vi "ConfigureChannels.vi"(8 "error in (no error)":errorcluster, 11 "Infiniium in":refnum<class "Infiniium.lvclass">) -> (0 "error out":errorcluster, 3 "Infiniium out":refnum<class "Infiniium.lvclass">)   [LabVIEW 2018, in "ScopePlugins.lvlib" / "Infiniium.lvclass"]
uses:
  Infiniium.lvclass
  Y:/Projects/PMUCal/Modules/Scope/ScopePlugins/ScopePluginBaseClass/ScopePluginsBase.lvclass
  ScopePluginBaseClass/ScopePluginsBase.lvclass/ScopePluginsBase.ctl
  ScopePluginBaseClass/Accessors/Read Handle.vi
  ScopePluginBaseClass/Accessors/Read Channels.vi
  ScopePluginBaseClass/Accessors/Read Connected.vi
  <vilib>/Utility/error.llb/Error Cluster From Error Code.vi
  <vilib>/ErrorRing/Error Ring.xnode
  <instrlib>/Agilent 90000 Series/Agilent 90000 Series.lvlib
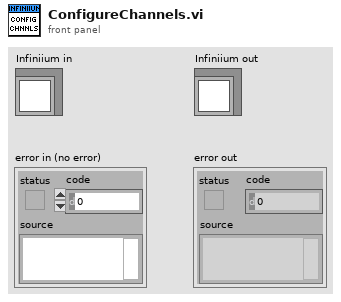
[diagram p1: front panel]
types:
  T1 = typedef "ScopePlugins.lvlib/Channels.ctl" = cluster{"Count":i32, "ChannelArray":T2[]}
  T2 = typedef "ScopePlugins.lvlib/Channel.ctl" = cluster{"Enabled":bool, "Name":string, "InputImpedance":dbl, "InputFreqMax":dbl, "ProbeAttn":dbl, "Coupling":enum16{"AC", "DC", "GND"}, "Offset":dbl, "Range":dbl, "Handle":string, "Connected":bool}
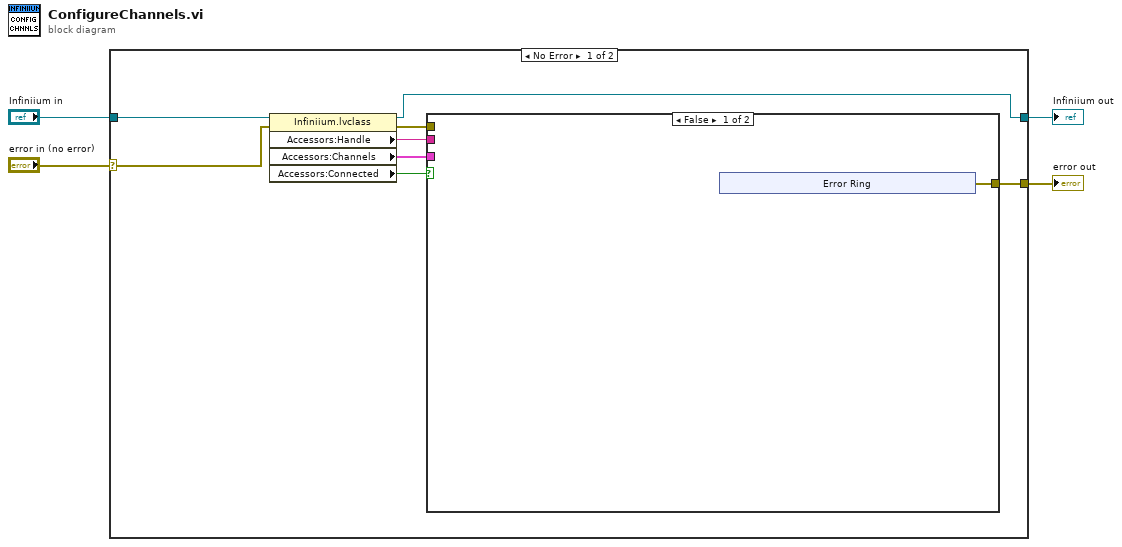
[diagram p0: block diagram]
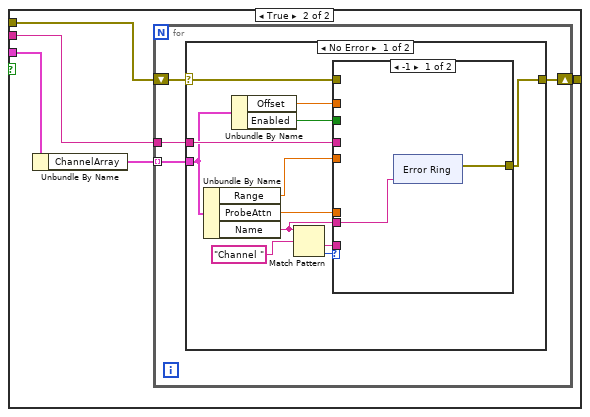
[diagram p2: hidden frame]
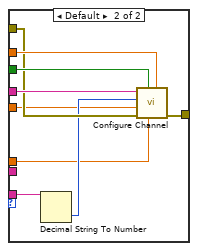
[diagram p3: hidden frame]
diagram:
  n1 = case shown="No Error" "error in (no error)" {
    selector: "error in (no error)" -> [w11 w59]
    tunnel: "Infiniium in" -> [w12 w60]
    tunnel: [w7 w60] -> w2
    tunnel: [w6 w59] -> w1
    frame No Error {
      n2 = property class="Infiniium.lvclass"(reference=w12, error in=w11) -> (reference out=w7:refnum<class "Infiniium.lvclass">, error out=w8:errorcluster, "Accessors:Handle"=w10:string, "Accessors:Channels"=w9:T1, "Accessors:Connected"=w5:bool)
      n3 = case shown="False" w5 {
        tunnel: w10 -> [_ w23]
        tunnel: w9 -> [_ w22]
        tunnel: w8 -> [_ w20]
        tunnel: [w13 w19] -> w6
        frame False {
          n4 = xnode "Error Ring"() -> ("error out"=w13:errorcluster)
        }
        frame True {
          n5 = Unbundle By Name(w22) -> ("ChannelArray"=w21:T2[])
          n6 = for {
            tunnel: w23 -> [w27]
            tunnel: w21 -> [w26] mode=indexing
            shift-right: [w24] -> w19
            shift-left: w20 -> [w25]
            n7 = case shown="No Error" w25 {
              selector: w25 -> [w34 w58]
              tunnel: w27 -> [w39 _]
              tunnel: w26 -> [w36 _]
              tunnel: [w32 w58] -> w24
              frame No Error {
                n8 = Unbundle By Name(w36) -> ("Range"=w29:dbl, "ProbeAttn"=w30:dbl, "Name"=w28:string)
                n9 = Unbundle By Name(w36) -> ("Offset"=w37:dbl, "Enabled"=w38:bool)
                n10 = Match Pattern(string=w28, regular expression="Channel ") -> (after substring=w31:string, offset past match=w33:i32)  [unwired: 1 in, 2 out]
                n11 = case shown="-1" w33 {
                  tunnel: w39 -> [_ w57]
                  tunnel: w38 -> [_ w56]
                  tunnel: w37 -> [_ w55]
                  tunnel: w34 -> [_ w54]
                  tunnel: [w41 w53] -> w32
                  tunnel: w31 -> [_ w52]
                  tunnel: w30 -> [_ w50]
                  tunnel: w29 -> [_ w49]
                  tunnel: w28 -> [w40 _]
                  frame -1 {
                    n12 = xnode "Error Ring"("parameter 0"=w40) -> ("error out"=w41:errorcluster)
                  }
                  frame Default {
                    n13 = Decimal String To Number(string=w52) -> (number=w51:i32)  [unwired: 2 in, 1 out]
                    n14 = call <instrlib>:"Configure Channel.vi"("Vertical Offset (0.0 V)"=w55, "Probe Attenuation (1.0)"=w50, "Enable Channel (T: Enable)"=w56, "error in (no error)"=w54, "Vertical Range (2.0 V)"=w49, "Channel (1: Channel 1)"=w51, "VISA resource name"=w57) -> ("error out"=w53:errorcluster)  [unwired: 3 in, 1 out]
                  }
                }
              }
              frame Error {
              }
            }
          }
        }
      }
    }
    frame Error {
    }
  }
  "error out" <- w1
  "Infiniium out" <- w2
